vi "CMC温度读取.vi"(8 "error in":errorcluster caption="错误输入", 11 "Channel":u16=81 format="%.0x") -> (0 "error out":errorcluster caption="错误输出", 2 "CMC1温度":i32[](array[numeric]), 3 "CMC2温度":i32[](array[numeric]))   [LabVIEW 2020]
uses:
  D/Program Files (x86)/National Instruments/LabVIEW 2020/user.lib/PCANBasic/PCANBasic.lvlib
panel:
  out "function return 2":u32 format="%.0x"
  out "function return 3":u32 format="%.0x"
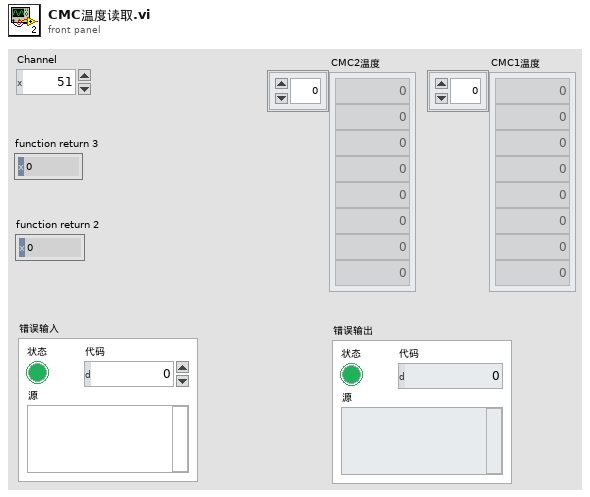
[diagram p1: front panel]
types:
  T1 = cluster{"ID":u32, "MSGTYPE":u8, "DLC":u8, "DATA[0]":u8, "DATA[1]":u8, "DATA[2]":u8, "DATA[3]":u8, "DATA[4]":u8, "DATA[5]":u8, "DATA[6]":u8, "DATA[7]":u8, "DATA[8]":u8, "DATA[9]":u8, "DATA[10]":u8, "DATA[11]":u8, "DATA[12]":u8, "DATA[13]":u8, "DATA[14]":u8, "DATA[15]":u8, "DATA[16]":u8, "DATA[17]":u8, "DATA[18]":u8, "DATA[19]":u8, "DATA[20]":u8, "DATA[21]":u8, "DATA[22]":u8, "DATA[23]":u8, "DATA[24]":u8, "DATA[25]":u8, "DATA[26]":u8, "DATA[27]":u8, "DATA[28]":u8, "DATA[29]":u8, "DATA[30]":u8, "DATA[31]":u8, "DATA[32]":u8, "DATA[33]":u8, "DATA[34]":u8, "DATA[35]":u8, "DATA[36]":u8, "DATA[37]":u8, "DATA[38]":u8, "DATA[39]":u8, "DATA[40]":u8, "DATA[41]":u8, "DATA[42]":u8, "DATA[43]":u8, "DATA[44]":u8, "DATA[45]":u8, "DATA[46]":u8, "DATA[47]":u8, "DATA[48]":u8, "DATA[49]":u8, "DATA[50]":u8, "DATA[51]":u8, "DATA[52]":u8, "DATA[53]":u8, "DATA[54]":u8, "DATA[55]":u8, "DATA[56]":u8, "DATA[57]":u8, "DATA[58]":u8, "DATA[59]":u8, "DATA[60]":u8, "DATA[61]":u8, "DATA[62]":u8, "DATA[63]":u8}
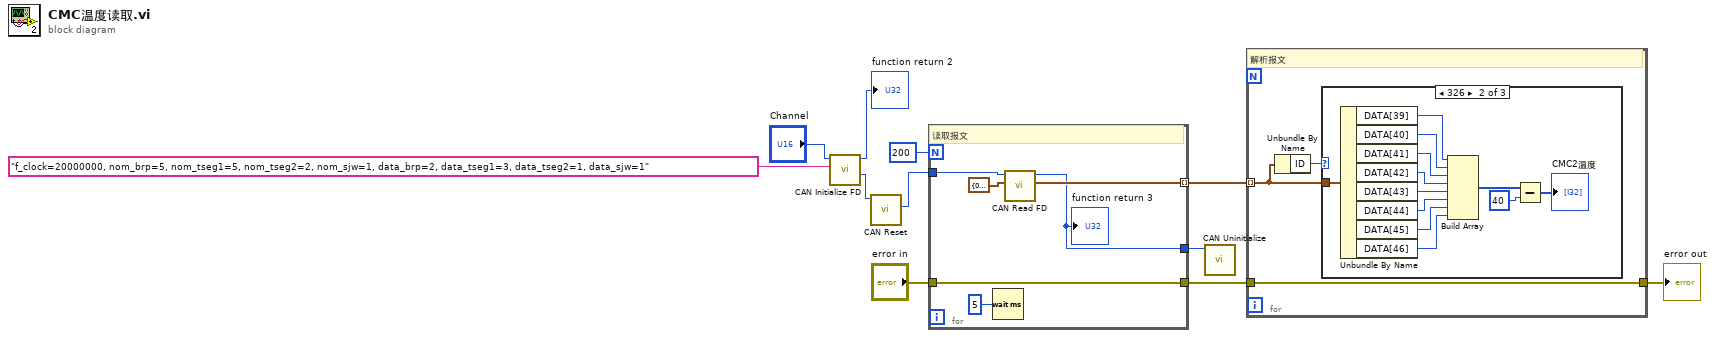
[diagram p0: block diagram]
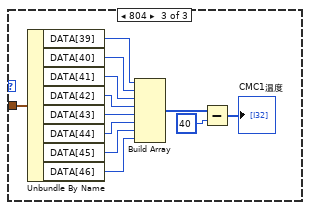
[diagram p3: hidden frame]
diagram:
  n1 = call "CAN Initialize FD.vi"("BitrateFD"="f_clock=20000000, nom_brp=5, nom_tseg1=5, nom_tseg2=2, nom_sjw=1, data_brp=2, data_tseg1=3, data_tseg2=1, data_sjw=1", "Channel"="Channel") -> ("Channel out"=w2:u16, "function return"=→"function return 2":u32)  [unwired: 7 in, 1 out]
  n2 = call "CAN Reset.vi"("Channel in"=w2) -> ("Channel out"=w1:u16)  [unwired: 9 in, 1 out]
  n3 = for {
    N: 200 -> [_]
    tunnel: [w16] -> w10 mode=indexing
    tunnel: [w14] -> w6
    tunnel: "error in" -> [w13]
    tunnel: [w13] -> w4
    tunnel: w1 -> [w12]
    # "读取报文"
    n4 = Wait (ms)(milliseconds to wait=u32 5 ("等待时间（毫秒）")) -> ()  [unwired: 1 out]
    n5 = call "CAN Read FD.vi"("MessageBuffer"=T1 {"ID"=0, "MSGTYPE"=0, "DLC"=0, "DATA[0]"=0, "DATA[1]"=0, "DATA[2]"=0, "DATA[3]"=0, "DATA[4]"=0, "DATA[5]"=0, "DATA[6]"=0, "DATA[7]"=0, "DATA[8]"=0, "DATA[9]"=0, "DATA[10]"=0, "DATA[11]"=0, "DATA[12]"=0, "DATA[13]"=0, "DATA[14]"=0, "DATA[15]"=0, "DATA[16]"=0, "DATA[17]"=0, "DATA[18]"=0, "DATA[19]"=0, "DATA[20]"=0, "DATA[21]"=0, "DATA[22]"=0, "DATA[23]"=0, "DATA[24]"=0, "DATA[25]"=0, "DATA[26]"=0, "DATA[27]"=0, "DATA[28]"=0, "DATA[29]"=0, "DATA[30]"=0, "DATA[31]"=0, "DATA[32]"=0, "DATA[33]"=0, "DATA[34]"=0, "DATA[35]"=0, "DATA[36]"=0, "DATA[37]"=0, "DATA[38]"=0, "DATA[39]"=0, "DATA[40]"=0, "DATA[41]"=0, "DATA[42]"=0, "DATA[43]"=0, "DATA[44]"=0, "DATA[45]"=0, "DATA[46]"=0, "DATA[47]"=0, "DATA[48]"=0, "DATA[49]"=0, "DATA[50]"=0, "DATA[51]"=0, "DATA[52]"=0, "DATA[53]"=0, "DATA[54]"=0, "DATA[55]"=0, "DATA[56]"=0, "DATA[57]"=0, "DATA[58]"=0, "DATA[59]"=0, "DATA[60]"=0, "DATA[61]"=0, "DATA[62]"=0, "DATA[63]"=0}, "Channel"=w12) -> ("MessageBuffer out"=w16:T1, "function return"=w14:u32)  [unwired: 6 in, 2 out]
    "function return 3" <- w14
  }
  n6 = call "CAN Uninitialize.vi"("Channel"=w6) -> ()  [unwired: 10 in, 1 out]
  n7 = for {
    tunnel: w10 -> [w19] mode=indexing
    tunnel: w4 -> [w18]
    tunnel: [w18] -> w3
    # "解析报文"
    n8 = Unbundle By Name(w19) -> ("ID"=w20:u32)
    n9 = case shown="326" w20 {
      tunnel: w19 -> [_ w21 w44]
      frame 0, Default {
      }
      frame 806 {
        n10 = Unbundle By Name(w21) -> ("DATA[39]"=w32:u8, "DATA[40]"=w31:u8, "DATA[41]"=w30:u8, "DATA[42]"=w29:u8, "DATA[43]"=w28:u8, "DATA[44]"=w27:u8, "DATA[45]"=w26:u8, "DATA[46]"=w25:u8)
        n11 = Build Array(w32, w31, w30, w29, w28, w27, w26, w25) -> (w23:u8[])
        n12 = Subtract(x=w23, y=40) -> (x-y=→"CMC2温度":i32[])
      }
      frame 804 {
        n13 = Unbundle By Name(w44) -> ("DATA[39]"=w43:u8, "DATA[40]"=w42:u8, "DATA[41]"=w41:u8, "DATA[42]"=w40:u8, "DATA[43]"=w39:u8, "DATA[44]"=w38:u8, "DATA[45]"=w37:u8, "DATA[46]"=w36:u8)
        n14 = Build Array(w43, w42, w41, w40, w39, w38, w37, w36) -> (w34:u8[])
        n15 = Subtract(x=w34, y=40) -> (x-y=→"CMC1温度":i32[])
      }
    }
  }
  "error out" <- w3
